vi "Clear Loaded Commands.vi"(8 "error in (no error)":errorcluster, 11 "Command Handler in":refnum<class "Command Handler.lvclass">) -> (0 "error out":errorcluster, 3 "Command Handler out":refnum<class "Command Handler.lvclass">)   [LabVIEW 2017, in "Command Handler.lvlib" / "Command Handler.lvclass"]
uses:
  Command Handler.lvclass
  Command Parents/Command.lvclass
  Command Handler.lvclass/Command Handler.ctl
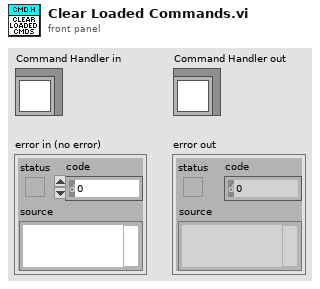
[diagram p1: front panel]
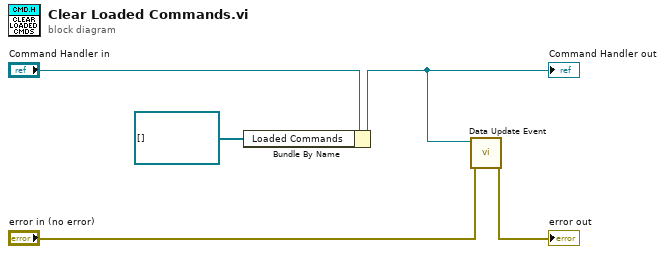
[diagram p0: block diagram]
diagram:
  n1 = Bundle By Name(cluster="Command Handler in", "Loaded Commands"=refnum<class "Command.lvclass">[] []) -> (w2:refnum<class "Command Handler.lvclass">)
  "Command Handler out" <- w2
  n2 = call "Data Update Event.vi"("error in (no error)"="error in (no error)", "Command Handler in"=w2) -> ("error out"=→"error out":errorcluster)  [unwired: 9 in]
